vi "fire1disc.vi"(11 "Reset Count":bool) -> (1 "Launcher State":T1, 3 "Done":bool)   [LabVIEW 2012]
uses:
  <vilib>/Rock Robotics/WPI/Solenoid/WPI_SolenoidValue.ctl
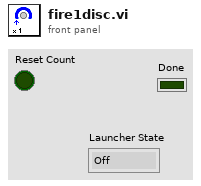
[diagram p1: front panel]
types:
  T1 = typedef "WPI_SolenoidValue.ctl" = enum16{"Off", "On", "Forward", "Reverse"}
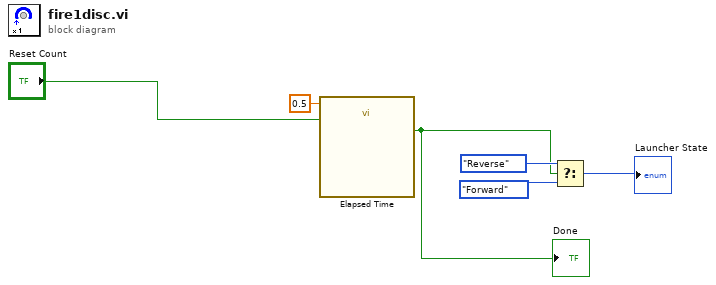
[diagram p0: block diagram]
diagram:
  n1 = call "Elapsed Time"("Time Target (s)"=0.5, "Reset"="Reset Count") -> ("Time has Elapsed"=w1:bool)  [unwired: 10 in, 7 out]
  "Done" <- w1
  n2 = Select(t=WPI_SolenoidValue."Reverse" ("Launcher State 2"), s=w1, f=WPI_SolenoidValue."Forward" ("Launcher State 2")) -> (s? t:f=→"Launcher State":T1)
